vi "Test golpi Package Installation.vi"() -> ()   [LabVIEW 2020, in "GOLPI library.lvlib"]
doc: "Only for testing of package installation.\n\n---\nGOLPI works only with lv_proc.dll library, which is part of vipm package or should be delivered together with packed library. Placement of this dll is selected in terminal of Start GNU Octave.vi."
uses:
  GOLPI library.lvlib
  Get Variable - polymorph parts/Get Double.vi
  Get Variable - polymorph parts/Get Struct.vi
panel:
  out "value":dbl format="%.2f"
  in  "quit":bool
  in  "what to test":enum16{"bitstream", "get struct"}(ring)
  in  "Cluster":cluster{"b":dbl, "c":string}
  out "read buffer 1":string
  in  "octave exe file or directory":path=path "C:/Program Files/GNU Octave/Octave-6.2.0/mingw64/bin/octave.bat"
  out "GNU Octave version":string
  out "exit code":i32
  out "error out":errorcluster
  out "pkg list after":string
  in  "working directory":path=path "C:/Users/labina/Documents"
  # "What it does:\n\nUninstall package\nSets bitstream/struct transfer\nChecks installed packages"
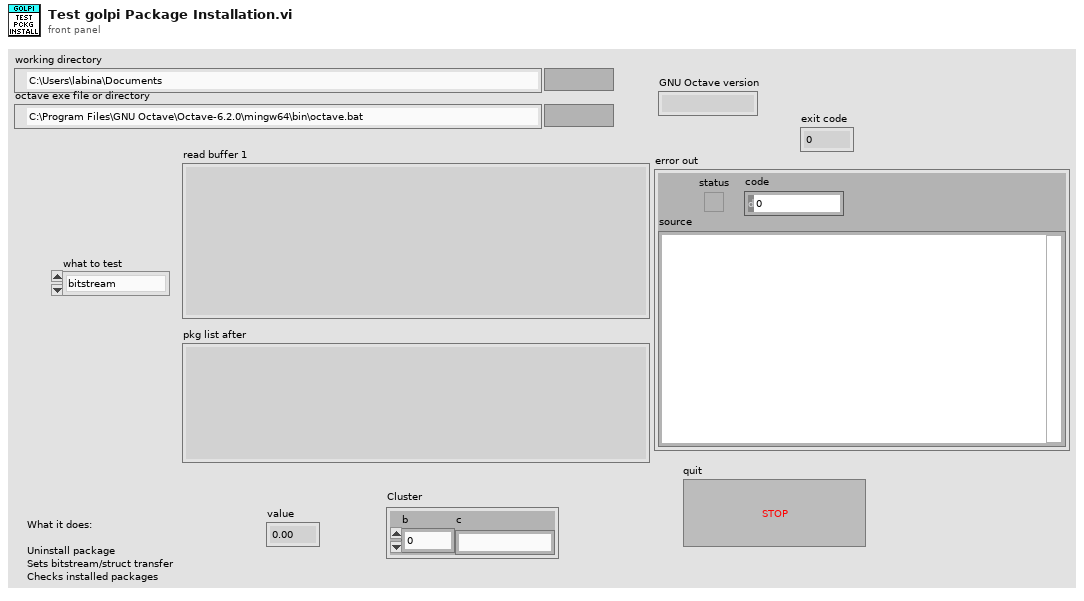
[diagram p1: front panel]
types:
  T1 = typedef "GOLPI library.lvlib/GOLPI reference Type Def.ctl" = cluster{"pipe handle":T2, "fast read timeout [ms]":u32, "fast read settle time [ms]":u32, "fast read to multiple [ms]":u32, "max elements per input line":u32, "slow read timeout [ms]":u32, "stdin double format specifier":string, "max elements per stdout output column":u32, "console mode bitstream":bool, "bitstream first read timeout [ms]":u32, "bitstream read timeout [ms]":u32, "struct transfer possible":bool, "matlab mode":bool}
  T2 = typedef "LV Process library.lvlib/Pipe Handle.ctl" = cluster{"lv_proc.dll file path":path, "process instance handle":u32[], "debug mode":bool, "debug data":cluster{"time":timestamp, "stdin":bool, "data":string}[]}
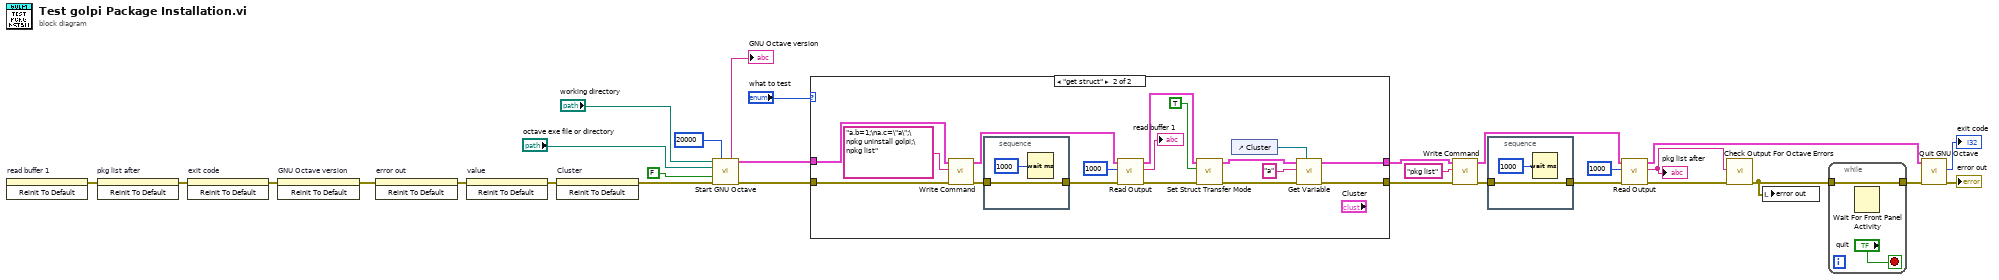
[diagram p0: block diagram]
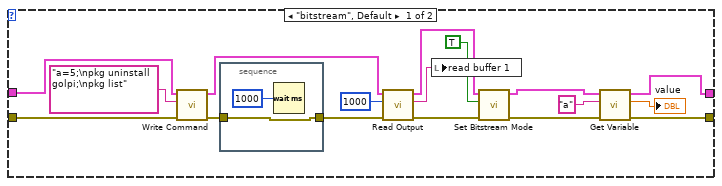
[diagram p2: hidden frame]
diagram:
  n1 = invoke on="read buffer 1" class="Str" method="Reinit To Default"() -> (error out=w2:errorcluster)  [unwired: 3 in, 2 out]
  n2 = invoke on="pkg list after" class="Str" method="Reinit To Default"(error in=w2) -> (error out=w1:errorcluster)  [unwired: 2 in, 2 out]
  n3 = invoke on="exit code" class="DigNum (strict)" method="Reinit To Default"(error in=w1) -> (error out=w4:errorcluster)  [unwired: 2 in, 2 out]
  n4 = invoke on="GNU Octave version" class="Str" method="Reinit To Default"(error in=w4) -> (error out=w5:errorcluster)  [unwired: 2 in, 2 out]
  n5 = invoke on="error out" class="Clust (strict)" method="Reinit To Default"(error in=w5) -> (error out=w6:errorcluster)  [unwired: 2 in, 2 out]
  n6 = invoke on="value" class="DigNum (strict)" method="Reinit To Default"(error in=w6) -> (error out=w7:errorcluster)  [unwired: 2 in, 2 out]
  n7 = invoke on="Cluster" class="Clust (strict)" method="Reinit To Default"(error in=w7) -> (error out=w3:errorcluster)  [unwired: 2 in, 2 out]
  n8 = call "Start GNU Octave.vi"("working directory"="working directory", "full start timeout [ms] (20000)"=u32 20000 ("Full start timeout [ms] (5000)"), "octave exe file or directory"="octave exe file or directory", "hide debug console (T)"=FALSE, "error in"=w3) -> ("GNU Octave version"=→"GNU Octave version":string, "GOLPI ref. out"=w14:T1, "error out"=w15:errorcluster)  [unwired: 7 in, 1 out]
  n9 = case shown="\"get struct\"" "what to test" {
    tunnel: w15 -> [w38 w63]
    tunnel: w14 -> [w39 w61]
    tunnel: [w33 w57] -> w12
    tunnel: [w32 w54] -> w11
    frame "bitstream", Default {
      n10 = call "Write Command.vi"("error in"=w38, "command"="a=5;\npkg uninstall golpi;\npkg list" ("command 1"), "GOLPI ref. in"=w39) -> ("error out"=w43:errorcluster, "GOLPI ref. out"=w42:T1)  [unwired: 7 in]
      n11 = stacked-sequence {
        tunnel: [w47] -> w44
        tunnel: w43 -> [w47]
        frame #0 {
          n12 = Wait (ms)(milliseconds to wait=u32 1000) -> ()  [unwired: 1 out]
        }
      }
      n13 = call "Read Output.vi"("error in"=w44, "byte count"=1000, "GOLPI ref. in"=w42) -> ("error out"=w46:errorcluster, "read buffer"=w37:string, "GOLPI ref. out"=w45:T1)  [unwired: 5 in, 1 out]
      n14 = local write "read buffer 1"(w37) -> ()
      n15 = call "Set Bitstream Mode.vi"("error in"=w46, "Bitstream mode (F)"=TRUE, "GOLPI ref. in"=w45) -> ("error out"=w35:errorcluster, "GOLPI ref. out"=w34:T1)  [unwired: 7 in]
      n16 = call-poly "Get Variable.vi"("error in"=w35, "variable name"="a", "GOLPI ref. in"=w34) -> ("error out"=w32:errorcluster, "value"=→"value":dbl, "GOLPI ref. out"=w33:T1)  [unwired: 6 in]
    }
    frame "get struct" {
      n17 = call "Write Command.vi"("error in"=w63, "command"="a.b=1;\na.c=\"a\";\npkg uninstall golpi;\npkg list" ("command 1"), "GOLPI ref. in"=w61) -> ("error out"=w64:errorcluster, "GOLPI ref. out"=w62:T1)  [unwired: 7 in]
      n18 = stacked-sequence {
        tunnel: [w66] -> w65
        tunnel: w64 -> [w66]
        frame #0 {
          n19 = Wait (ms)(milliseconds to wait=u32 1000) -> ()  [unwired: 1 out]
        }
      }
      n20 = call "Read Output.vi"("error in"=w65, "byte count"=1000, "GOLPI ref. in"=w62) -> ("error out"=w51:errorcluster, "read buffer"=→"read buffer 1":string, "GOLPI ref. out"=w53:T1)  [unwired: 5 in, 1 out]
      n21 = call "Set Struct Transfer Mode.vi"("error in"=w51, "Allow struct tranfer (False)"=TRUE, "GOLPI ref. in"=w53) -> ("error out"=w50:errorcluster, "GOLPI ref. out"=w52:T1)  [unwired: 6 in, 1 out]
      n22 = control-ref of="Cluster"() -> (w55:refnum<vi>)
      n23 = call-poly "Get Variable.vi"("cluster ref (empty)"=w55, "error in"=w50, "variable"="a", "GOLPI ref in"=w52) -> ("error out"=w54:errorcluster, "GOLPI ref. out"=w57:T1)  [unwired: 5 in, 1 out]
    }
  }
  n24 = call "Write Command.vi"("error in"=w11, "command"="pkg list", "GOLPI ref. in"=w12) -> ("error out"=w26:errorcluster, "GOLPI ref. out"=w28:T1)  [unwired: 7 in]
  n25 = stacked-sequence {
    tunnel: [w68] -> w25
    tunnel: w26 -> [w68]
    frame #0 {
      n26 = Wait (ms)(milliseconds to wait=u32 1000) -> ()  [unwired: 1 out]
    }
  }
  n27 = call "Read Output.vi"("error in"=w25, "byte count"=1000, "GOLPI ref. in"=w28) -> ("error out"=w18:errorcluster, "read buffer"=w19:string, "GOLPI ref. out"=w27:T1)  [unwired: 5 in, 1 out]
  "pkg list after" <- w19
  n28 = call "Check Output For Octave Errors.vi"("error in"=w18, "read buffer"=w19) -> ("error out"=w8:errorcluster)  [unwired: 9 in]
  n29 = local write "error out"(w8) -> ()
  n30 = while {
    tunnel: [w70] -> w9
    tunnel: w8 -> [w70]
    stop <- "quit" stop-if-true
    n31 = Wait For Front Panel Activity() -> ()  [unwired: 3 in, 1 out]
  }
  n32 = call "Quit GNU Octave.vi"("error in"=w9, "GOLPI ref. in"=w27) -> ("error out"=→"error out":errorcluster, "exit code"=→"exit code":i32)  [unwired: 8 in]
